vi "PriorityToBufferIndex.vi"(10 "number of buffers":i32, 11 "priority":i32) -> (0 "lowest priority?":bool, 1 "highest priority?":bool, 2 "buffer index":i32, 3 "priority out":i32)   [LabVIEW 2013, in "CLM_PriorityLocalMessage.lvclass"]
uses:
  CLM_PriorityLocalMessage.lvclass
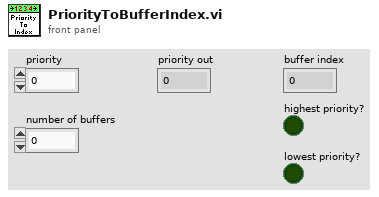
[diagram p1: front panel]
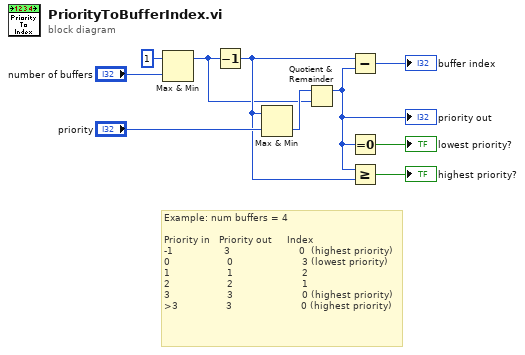
[diagram p0: block diagram]
diagram:
  # "Example: num buffers = 4\n\nPriority in   Priority out     Index\n-1                 3                       0  (highest priority)\n0                   0                       3 (lowest priority)\n1                   1                       2\n2                   2                       1\n3                   3                       0 (highest priority)\n>3                3                       0 (highest priority)"
  n1 = Max & Min(x=1, y="number of buffers") -> (max(x,y)=w1:i32)  [unwired: 1 out]
  n2 = Decrement(x=w1) -> (x-1=w5:i32)
  n3 = Max & Min(x=w5, y="priority") -> (min(x,y)=w9:i32)  [unwired: 1 out]
  n4 = Quotient & Remainder(x=w9, y=w1) -> (x-y*floor(x/y)=w6:i32)  [unwired: 1 out]
  "priority out" <- w6
  n5 = Subtract(x=w5, y=w6) -> (x-y=→"buffer index":i32)
  n6 = Equal To 0?(x=w6) -> (x = 0?=→"lowest priority?":bool)
  n7 = Greater Or Equal?(x=w6, y=w5) -> (x >= y?=→"highest priority?":bool)
